vi "Server VI or RT.vi"() -> ()   [LabVIEW 2013]
panel:
  in  "remote port":u16=3363
  in  "address":string="169.254.82.40"
  out "error out":errorcluster
  out "bytes written":i32
  in  "data in":string
  in  "Stop Button":bool
  # "RT or Server VI"
  # "Note : \n\n1. Mention the Client Address and port no before running the  VI"
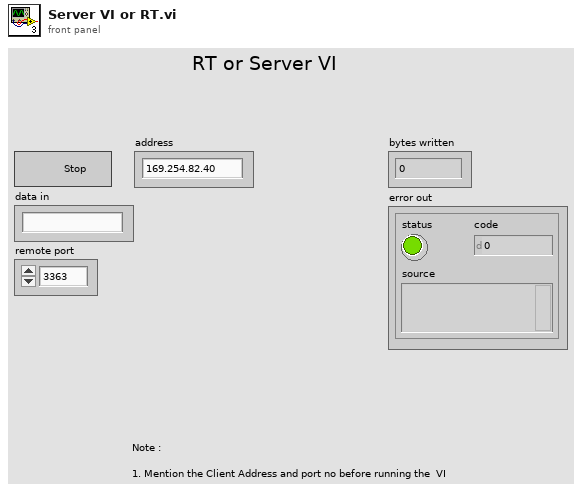
[diagram p1: front panel]
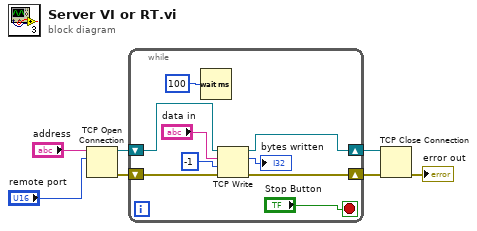
[diagram p0: block diagram]
diagram:
  n1 = TCP Open Connection(address="address", remote port or service name="remote port") -> (connection ID=w7:refnum<k5>, error out=w5:errorcluster)  [unwired: 3 in]
  n2 = while {
    shift-right: [w15] -> w6
    shift-left: w7 -> [w16]
    shift-right: [w13] -> w4
    shift-left: w5 -> [w14]
    stop <- "Stop Button" stop-if-true
    n3 = Wait (ms)(milliseconds to wait=u32 100) -> ()  [unwired: 1 out]
    n4 = TCP Write(connection ID=w16, data in="data in", error in (no error)=w14, 9:-1 ("timeout ms (25000)")) -> (connection ID out=w15:refnum<k5>, bytes written=→"bytes written":i32, error out=w13:errorcluster)
  }
  n5 = TCP Close Connection(connection ID=w6, error in (no error)=w4) -> (error out=→"error out":errorcluster)  [unwired: 1 in, 1 out]
